vi "libssh2_knownhost_get - with previous - returns next host.vi"() -> ()   [LabVIEW 2017, in "unit_tests.lvlib"]
uses:
  unit_tests.lvlib
  libssh2/Host Key Refnum.ctl
  libssh2/libssh2_init_default.vi
  libssh2/libssh2_session_init_ex.vi
  libssh2/libssh2.lvlib
  <vilib>/PNR/Transparent Assertions/Transparent Assertions/Transparent Assertions.lvlib
panel:
  out "error out":errorcluster
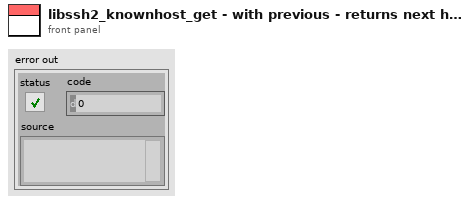
[diagram p1: front panel]
types:
  T1 = typedef "libssh2.lvlib/Host Key Refnum.ctl" = refnum<k1>
  T2 = typedef "libssh2.lvlib/Session Refnum.ctl" = refnum<k1>
  T3 = typedef "libssh2.lvlib/Host Key Database Refnum.ctl" = refnum<k1>
  T4 = typedef "libssh2.lvlib/libssh2_knownhost.ctl" = cluster{"magic":u32, "node":u64, "name":string, "key":string, "typemask":i32}
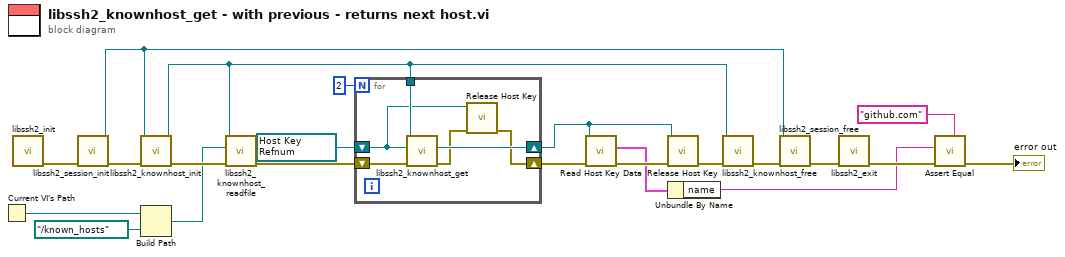
[diagram p0: block diagram]
diagram:
  w2 = T1 refnum items=["host key"] ("next")
  n1 = Current VI's Path() -> (path=w13:path)
  n2 = call-poly "libssh2_init.vi"() -> ("error out"=w21:errorcluster)  [unwired: 11 in]
  n3 = call "libssh2_session_init.vi"("error in (no error)"=w21) -> ("error out"=w20:errorcluster, "session"=w17:T2)  [unwired: 9 in]
  n4 = call "libssh2_knownhost_init.vi"("error in (no error)"=w20, "session"=w17) -> ("error out"=w15:errorcluster, "host key database"=w10:T3)  [unwired: 8 in]
  n5 = Build Path(base path=w13, name or relative path=path "../known_hosts" ("filename")) -> (appended path=w11:path)
  n6 = call "libssh2_knownhost_readfile.vi"("error in (no error)"=w15, "filename"=w11, "host key database"=w10) -> ("error out"=w14:errorcluster)  [unwired: 7 in, 1 out]
  n7 = for {
    N: 2 -> [_]
    tunnel: w10 -> [w28]
    shift-right: [w27] -> w6
    shift-left: w2 -> [w25]
    shift-right: [w23] -> w8
    shift-left: w14 -> [w26]
    n8 = call "libssh2_knownhost_get.vi"("error in (no error)"=w26, "previous host key"=w25, "host key database"=w28) -> ("error out"=w24:errorcluster, "host key"=w27:T1)  [unwired: 6 in, 1 out]
    n9 = call "Release Host Key.vi"("error in (no error)"=w24, "host key"=w25) -> ("error out"=w23:errorcluster)  [unwired: 9 in]
  }
  n10 = call "Read Host Key Data.vi"("error in (no error)"=w8, "host key"=w6) -> ("error out"=w7:errorcluster, "host key data"=w5:T4)  [unwired: 8 in]
  n11 = call "Release Host Key.vi"("error in (no error)"=w7, "host key"=w6) -> ("error out"=w9:errorcluster)  [unwired: 9 in]
  n12 = Unbundle By Name(w5) -> ("name"=w4:string)
  n13 = call "libssh2_knownhost_free.vi"("error in (no error)"=w9, "host key database"=w10) -> ("error out"=w16:errorcluster)  [unwired: 9 in]
  n14 = call "libssh2_session_free.vi"("error in (no error)"=w16, "session"=w17) -> ("error out"=w19:errorcluster)  [unwired: 9 in]
  n15 = call "libssh2_exit.vi"("error in (no error)"=w19) -> ("error out"=w18:errorcluster)  [unwired: 10 in]
  n16 = call <vilib>:"Assert Equal.vi"("Expected"="github.com" ("key"), "error in (no error)"=w18, "Actual"=w4) -> ("error out"=→"error out":errorcluster)  [unwired: 8 in]
